vi "Parse XML Heap.vi"(8 "error in (no error)":errorcluster, 10 "Root Parent":string, 11 "XML":string) -> (0 "error out":errorcluster, 3 "Items":refnum<class "Data Item.lvclass">[](array[class]))   [LabVIEW 2026, in "VILab.lvlib"]
uses:
  VILab.lvlib
  Classes/Data Item/Data Item.lvclass
  <vilib>/xml/Load XML String.vi
  <vilib>/xml/Close Reference(Node).vi
  <vilib>/xml/NI_XML.lvlib
  <resource>/objmgr/DOMUserDefRef.rc
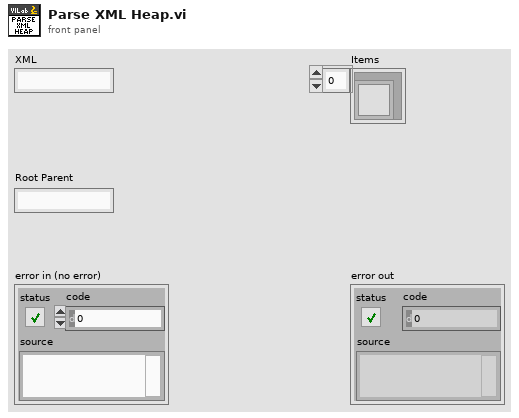
[diagram p1: front panel]
types:
  T1 = cluster{"DocumentElement":refnum<k20>, "Root Parent":string, i32}
  T2 = cluster{"DocumentElement":refnum<k20>, "Root Parent":string, i32}[]
  T3 = cluster{refnum<k20>, "Accessors:Item ID":string, i32}
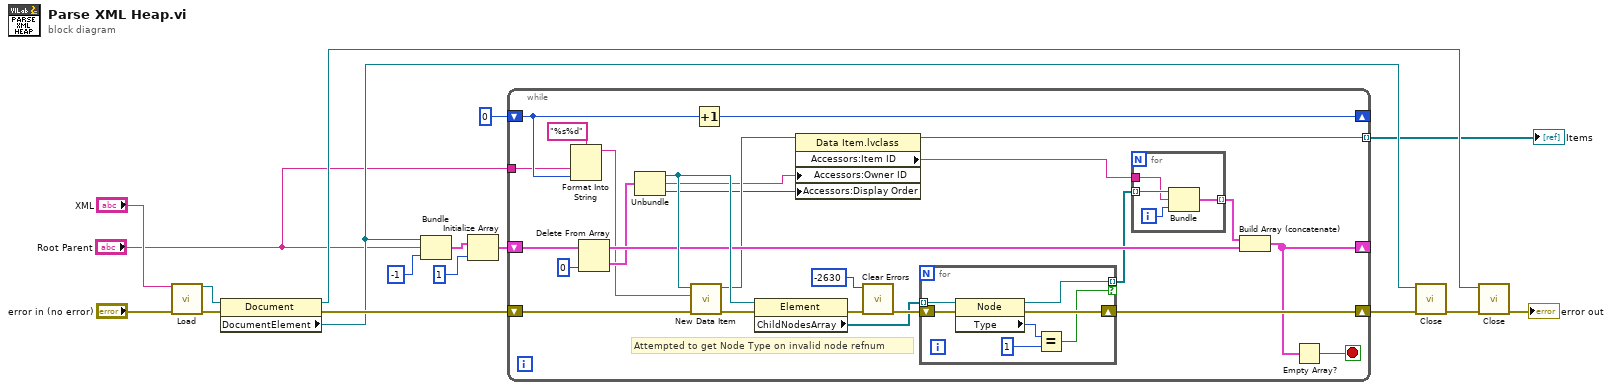
[diagram p0: block diagram]
diagram:
  n1 = call-poly <vilib>:"Load.vi"("XML string"="XML", "error in (no error)"="error in (no error)") -> ("DOM document out"=w11:refnum<k20>, "error out"=w17:errorcluster)  [unwired: 11 in, 1 out]
  n2 = property class="Document"(reference=w11, error in=w17) -> (reference out=w10:refnum<k20>, error out=w16:errorcluster, "DocumentElement"=w9:refnum<k20>)
  n3 = Bundle("DocumentElement"=w9, "Root Parent"="Root Parent", -1) -> (w5:T1)  [unwired: 1 in]
  n4 = Initialize Array(w5, 1 ("dimension size")) -> (w3:T2)
  n5 = while {
    shift-right: [w39] -> w14
    shift-left: w16 -> [w40]
    shift-right: [w34] -> _
    shift-left: w3 -> [w37]
    tunnel: [w26] -> w6 mode=indexing
    shift-right: [w19] -> _
    shift-left: 0 -> [w22]
    tunnel: "Root Parent" -> [w18]
    stop <- w33 stop-if-true
    # "Attempted to get Node Type on invalid node refnum"
    n6 = Format Into String(format string="%s%d", w18, w22) -> (resulting string=w20:string)  [unwired: 2 in, 1 out]
    n7 = Delete From Array(array=w37, index=0) -> (deleted portion=w31:T1, array with subset deleted=w36:T2)  [unwired: 1 in]
    n8 = Unbundle(w31) -> ("DocumentElement"=w38:refnum<k20>, "Root Parent"=w24:string, w23:i32)
    n9 = call "New Data Item.vi"("error in (no error)"=w40, "Item ID"=w20, "node in"=w38) -> ("error out"=w41:errorcluster, "Data Item"=w30:refnum<class "Data Item.lvclass">)  [unwired: 7 in]
    n10 = Increment(x=w22) -> (x+1=w19:i32)
    n11 = property class="Element"(reference=w38, error in=w41) -> (error out=w43:errorcluster, "ChildNodesArray"=w32:refnum<k20>[])  [unwired: 1 out]
    n12 = property class="Data Item.lvclass"(reference=w30, "Accessors:Owner ID"=w24, "Accessors:Display Order"=w23) -> (reference out=w26:refnum<class "Data Item.lvclass">, "Accessors:Item ID"=w25:string)  [unwired: 1 in, 1 out]
    n13 = call <vilib>:"Clear Errors.vi"("error in (no error)"=w43, "specific error code to clear (0: all)"=-2630) -> ("error out"=w42:errorcluster)  [unwired: 4 in, 1 out]
    n14 = for {
      shift-right: [w49] -> w39
      shift-left: w42 -> [w50]
      tunnel: w32 -> [w48] mode=indexing
      tunnel: [w47] -> w29 mode=indexing if=w44
      n15 = property class="Node"(reference=w48, error in=w50) -> (reference out=w47:refnum<k20>, error out=w49:errorcluster, "Type"=w46:i32)
      n16 = Equal?(x=w46, y=1) -> (x = y?=w44:bool)
    }
    n17 = for {
      tunnel: w29 -> [w54] mode=indexing
      tunnel: [w52] -> w28 mode=indexing
      tunnel: w25 -> [w51]
      i -> [w53]
      n18 = Bundle(w54, "Accessors:Item ID"=w51, w53) -> (w52:T3)  [unwired: 1 in]
    }
    n19 = Build Array (concatenate)(w28, w36) -> (w34:T2)
    n20 = Empty Array?(array=w34) -> (empty?=w33:bool)
  }
  "Items" <- w6
  n21 = call-poly <vilib>:"Close.vi"("error in (no error)"=w14, "node"=w9) -> ("error out"=w15:errorcluster)  [unwired: 7 in]
  n22 = call-poly <vilib>:"Close.vi"("error in (no error)"=w15, "node"=w10) -> ("error out"=→"error out":errorcluster)  [unwired: 7 in]
